vi "XYZStage-Conditional acknowledgement wait.vi"(8 "error in (no error)":errorcluster, 11 "XYZ Stage data to queue":T1={"Command"=enum."Dequeue", "Channel"="Z", "X"=0.0, "Y"=0.0, "Z"=0.0, "Speed"=0, "Zero"=FALSE, "Use acknowledgement?"=TRUE} {"Speed" format="Speed= %.0f"; "Z" format="Z= %#_g"; "Y" format="Y= %#_g"; "X" format="X= %#_g"}) -> (0 "error out":errorcluster, 1 "Timed out while waiting for acknowledgement":bool, 3 "Acknowledgement Message out":string)   [LabVIEW 2017]
uses:
  Typedefs/XYZ stage data.ctl
  Typedefs/XYZ stage states.ctl
  Typedefs/XYZ channel ring.ctl
  Typedefs/Command acknowledgment states.ctl
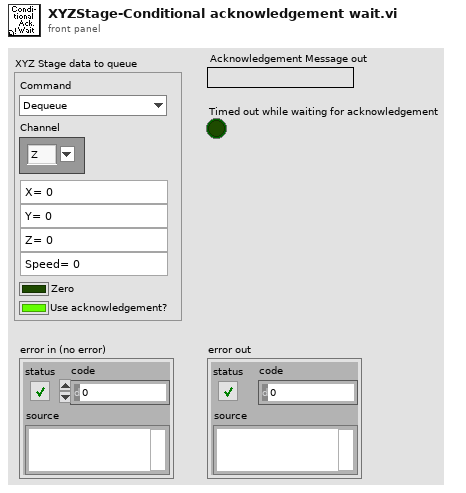
[diagram p1: front panel]
types:
  T1 = typedef "XYZ stage data.ctl" = cluster{"Command":T2, "Channel":T3, "X":sgl, "Y":sgl, "Z":sgl, "Speed":i32, "Zero":bool, "Use acknowledgement?":bool}
  T2 = typedef "XYZ stage states.ctl" = enum16{"Dequeue", "Initialize", "Read Position", "Read Speed Setting", "Move", "Set Max Speed", "Reset Axis", "Stop all movement"}
  T3 = typedef "XYZ channel ring.ctl" = string
  T4 = typedef "Command acknowledgment states.ctl" = enum16{"Acknowledge", "Wait for acknowledgment", "Release queue"}
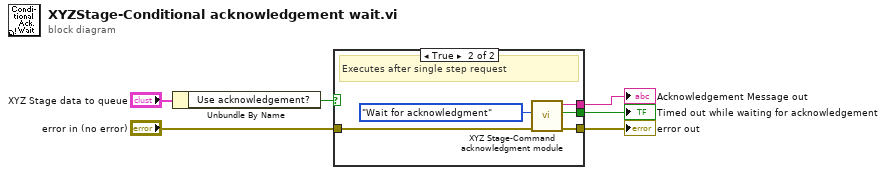
[diagram p0: block diagram]
diagram:
  n1 = Unbundle By Name("XYZ Stage data to queue") -> ("Use acknowledgement?"=w6:bool)
  n2 = case shown="True" w6 {
    tunnel: "error in (no error)" -> [w7 w11]
    tunnel: [w7 w10] -> w2
    tunnel: [_ w9] -> w3
    tunnel: [_ w8] -> w4
    frame False {
      # "Does not wait for an acknowledgement after a continuous movement request."
      # "Executes after continuous move request"
    }
    frame True {
      # "Executes after single step request"
      n3 = call "XYZ Stage-Command acknowledgment module.vi"("error in"=w11, "State"=Command_acknowledgment_states."Wait for acknowledgment") -> ("error out"=w10:errorcluster, "Timed out while waiting for acknowledgement"=w9:bool, "Acknowledgement Message out"=w8:string)  [unwired: 7 in]
    }
  }
  "Acknowledgement Message out" <- w4
  "Timed out while waiting for acknowledgement" <- w3
  "error out" <- w2
